vi "Wavform_Select dt and check valid time.vi"(8 "Use Merge Dt":bool, 10 "Waveform To Merge":T1, 11 "Waveform":T1) -> (1 "Selected Dt Out":dbl, 2 "Waveform To Merge":T1, 3 "Waveform":T1)   [LabVIEW 2020]
uses:
  Universal Controls/Waveform_Data.ctl
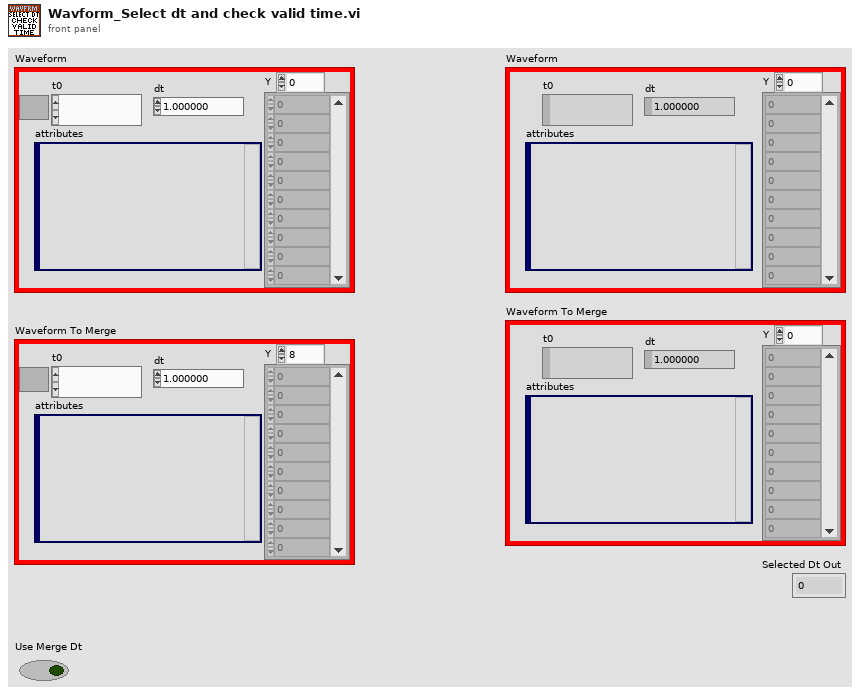
[diagram p1: front panel]
types:
  T1 = typedef "Waveform_Data.ctl" = waveform(dbl)
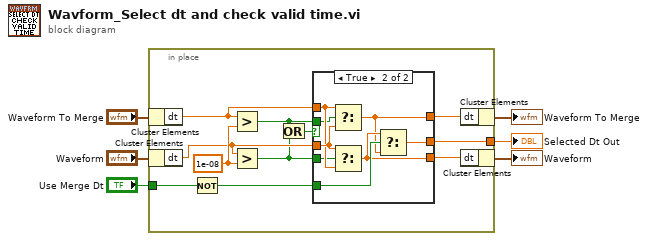
[diagram p0: block diagram]
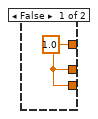
[diagram p2: hidden frame]
diagram:
  n1 = in-place {
    in-place-border: [w15] -> w4
    in-place-border: "Use Merge Dt" -> [w14]
    w17 = 1e-08 ("y")
    n2 = in-place-cluster #1("Waveform To Merge") -> ("dt"=w11:dbl)
    n3 = in-place-cluster #2("Waveform") -> ("dt"=w12:dbl)
    n4 = Not(x=w14) -> (.not. x?=w16:bool)
    n5 = Greater?(x=w11, y=w17) -> (0:w9:bool)
    n6 = Greater?(x=w12, y=w17) -> (0:w8:bool)
    n7 = Or(x=w9, y=w8) -> (x .or. y?=w7:bool)
    n8 = case shown="True" w7 {
      tunnel: w16 -> [_ w26]
      tunnel: [w18 w25] -> w15
      tunnel: [w18 w24] -> w13
      tunnel: w12 -> [_ w23]
      tunnel: w11 -> [_ w22]
      tunnel: [w18 w21] -> w10
      tunnel: w9 -> [_ w20]
      tunnel: w8 -> [_ w19]
      frame False {
        w18 = 1.0 ("dt")
      }
      frame True {
        n9 = Select(t=w22, s=w20, f=w23) -> (s? t:f=w21:dbl)
        n10 = Select(t=w23, s=w19, f=w22) -> (s? t:f=w24:dbl)
        n11 = Select(t=w24, s=w26, f=w21) -> (s? t:f=w25:dbl)
      }
    }
    n12 = in-place-cluster #1("dt"=w10) -> (→"Waveform To Merge":T1)
    n13 = in-place-cluster #2("dt"=w13) -> (→"Waveform":T1)
  }
  "Selected Dt Out" <- w4
